vi "常见错误连线示例.vi"() -> ()   [LabVIEW 2009]
panel:
  out "Slide":u8(slide) scale=0.0..100.0
  in  "Numeric 3":dbl
  out "String 4":string
  in  "String 3":string
  out "String 2":string
  in  "String":string
  out "Numeric 2":dbl
  in  "Boolean":bool
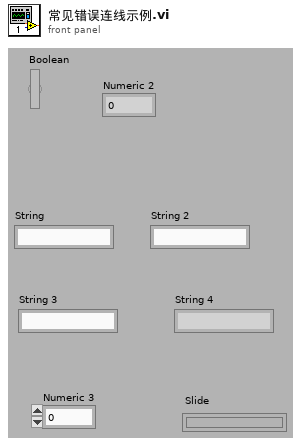
[diagram p1: front panel]
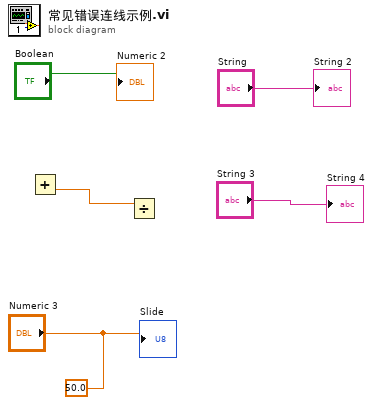
[diagram p0: block diagram]
diagram:
  w1 = 50.0 ("Numeric 3")
  n1 = Add() -> (y=w2:dbl)  [unwired: 1 in, 1 out]
  n2 = Divide(x=w2) -> ()  [unwired: 1 in, 1 out]
  "Numeric 2" <- "Boolean"
  "String 2" <- "String"
  "String 4" <- "String 3"
  "Slide" <- "Numeric 3"
